vi "YokoGS200 Get Limits.vi"(8 "error in (no error)":errorcluster, 11 "VISA Rsrc":refnum<visa-resource-name>="SR530") -> (0 "error out":errorcluster, 1 "VoltLimit":dbl caption="Voltage Limit", 2 "CurrLimit":dbl caption="Current Limit", 3 "VISA Rsrc Out":refnum<visa-resource-name>="GPIB0::12::INSTR")   [LabVIEW 2019]
panel:
  out "ChaineRep":string caption="Chaîne de réponse"
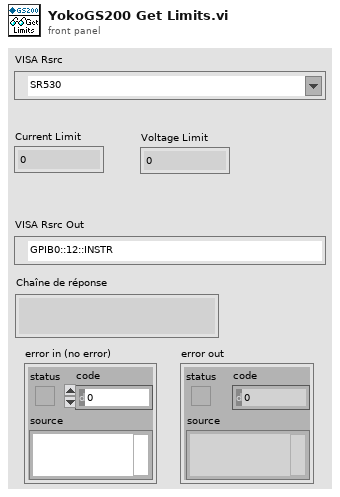
[diagram p1: front panel]
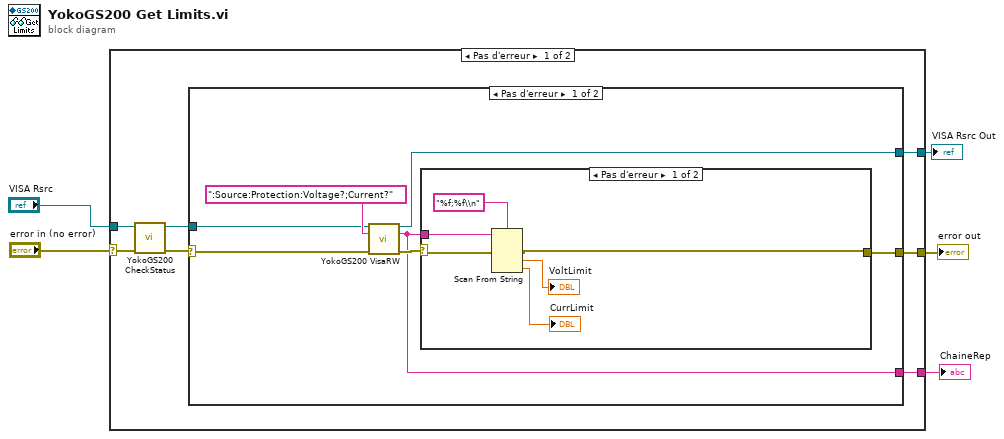
[diagram p0: block diagram]
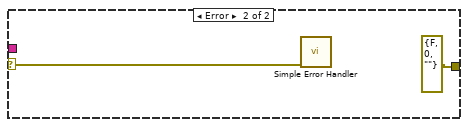
[diagram p2: hidden frame]
diagram:
  n1 = case shown="Pas d'erreur" "error in (no error)" {
    selector: "error in (no error)" -> [w8 w30]
    tunnel: "VISA Rsrc" -> [w9 w31]
    tunnel: [w11 w30] -> w4
    tunnel: [w12 w31] -> w3
    tunnel: [w10 _] -> w2
    frame No Error {
      n2 = call <userlib>:"YokoGS200 CheckStatus.vi"("error in (no error)"=w8, "VISA Rsrc"=w9) -> ("error out"=w6:errorcluster, "VISA Rsrc Out"=w7:refnum<visa-resource-name>)  [unwired: 6 in, 2 out]
      n3 = case shown="Pas d'erreur" w6 {
        selector: w6 -> [w13 w29]
        tunnel: [w19 w28] -> w12
        tunnel: [w16 w29] -> w11
        tunnel: [w15 _] -> w10
        tunnel: w7 -> [w14 w28]
        frame No Error {
          n4 = call <userlib>:"YokoGS200 VisaRW.vi"("VISA Rsrc"=w14, "ChaineCom"=":Source:Protection:Voltage?;Current?" ("string (\"\")"), "error in (no error)"=w13) -> ("VISA Rsrc Out"=w19:refnum<visa-resource-name>, "ChaineRep"=w15:string, "error out"=w17:errorcluster)  [unwired: 8 in, 2 out]
          n5 = case shown="Pas d'erreur" w17 {
            selector: w17 -> [w25 w26]
            tunnel: [w20 errorcluster {"status"=FALSE, "code"=0, "source"=""} ("error IO")] -> w16
            tunnel: w15 -> [w24 _]
            frame No Error {
              n6 = Scan From String(format string="%f;%f\\n", input string=w24, error in=w25) -> (error out=w20:errorcluster, output 1=→"VoltLimit":dbl, output 2=→"CurrLimit":dbl)  [unwired: 3 in, 2 out]
            }
            frame Error {
              n7 = call <vilib>:"Simple Error Handler.vi"("error in (no error)"=w26) -> ()  [unwired: 4 in, 5 out]
            }
          }
        }
        frame Error {
        }
      }
    }
    frame Error {
    }
  }
  "error out" <- w4
  "VISA Rsrc Out" <- w3
  "ChaineRep" <- w2
